vi "外控留样模式参数.vi"() -> ()   [LabVIEW 2016, in "超标留样集成.lvlib" / "德润DR803M超标留样.lvlib"]
uses:
  <vilib>/Utility/miscctls.llb/LVPointTypeDef.ctl
panel:
  out "读取更新":bool
  in  "返回":bool
  in  "模拟设置":bool
  in  "每瓶次数：":dbl
  in  "平行样：":dbl
  in  "每次留样：":dbl
  in  "留样瓶数：":dbl
  in  "当前瓶号：":dbl
  # "在该画面下，可设置该模式下的采样参数，包括当前瓶号、平行样、留样瓶数、每瓶次数和每次留样量。"
  # "mL"
  # "mg/L"
  # "COD\n模拟\n设置"
  # "mg/L"
  # "mg/L"
  # "mg/L"
  # "mg/L"
  # "氨氮\n模拟\n设置"
  # "mg/L"
  # "mg/L"
  # "mg/L"
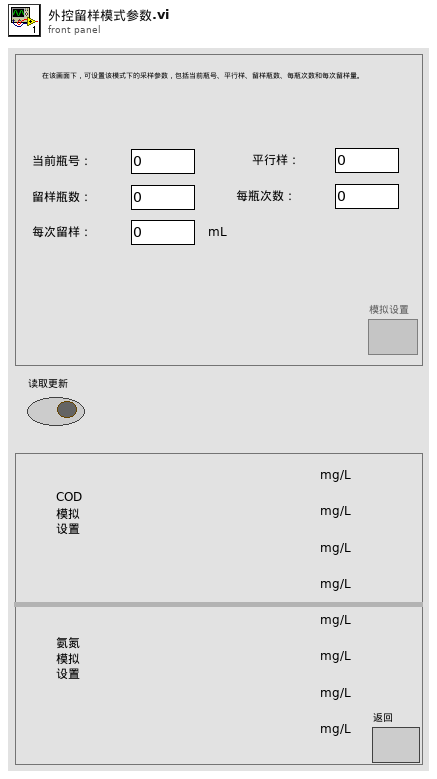
[diagram p1: front panel]
types:
  T1 = typedef "LVPointTypeDef.ctl" = cluster{"Horizontal":i16, "Vertical":i16}
  T2 = cluster{"当前瓶号：":dbl, "平行样：":dbl, "留样瓶数：":dbl, "每瓶次数：":dbl, "每次留样：":dbl}
  T3 = cluster{"采样器状态":enum16{"停止", "运行", "系统初始化-2", "系统初始化-3", "初始化失败"}, "仪器时间":timestamp, "留样结果":bool, "工作模式":u16, "当前瓶号":u16, "平行样数":u16, "采样瓶数":u16, "设定每瓶采样次数":u16, "每瓶采样量":u16, "当前进程":u16, "当前瓶已采次数":u16, "留样中":bool}
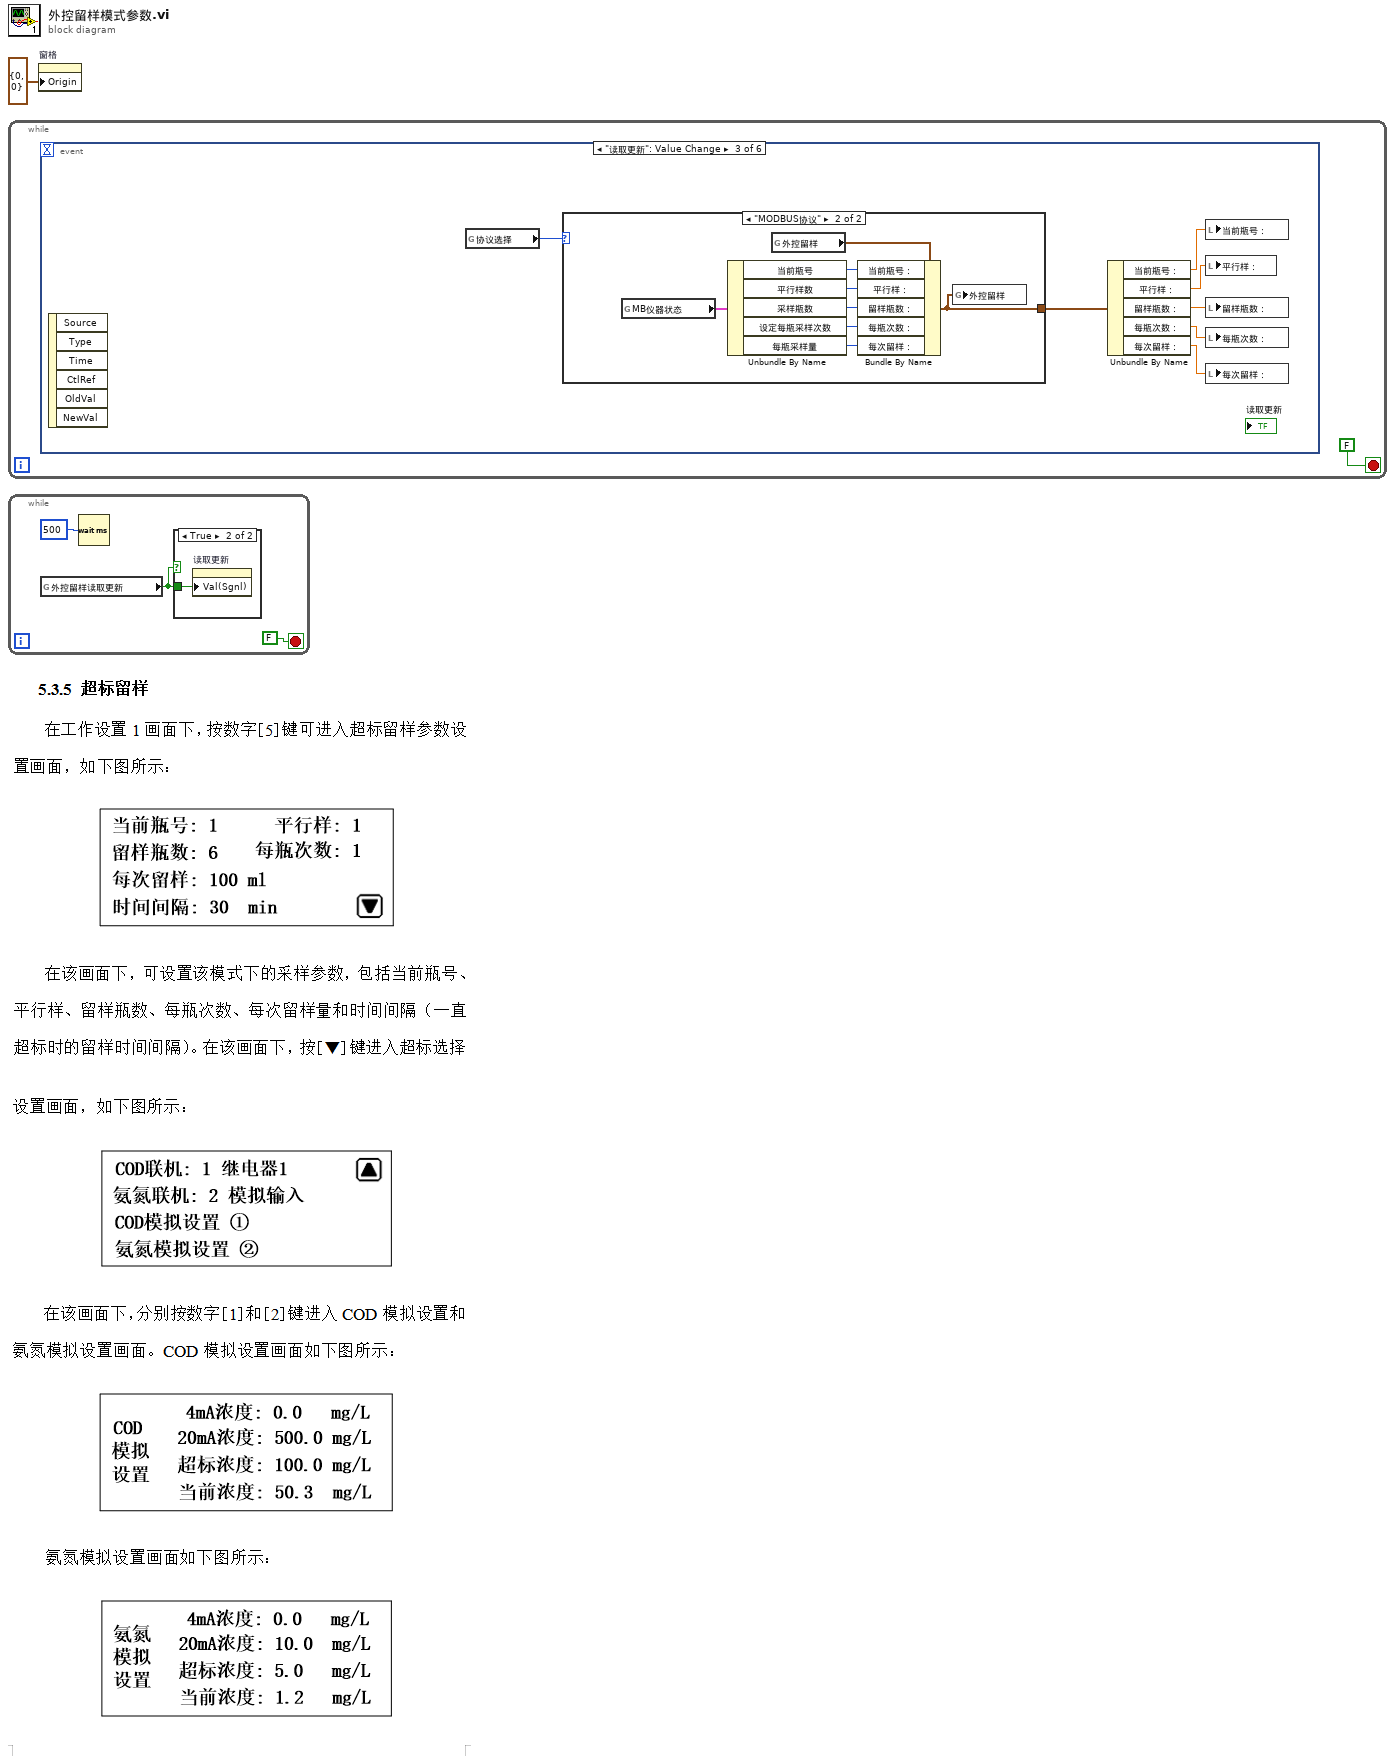
[diagram p0: block diagram]
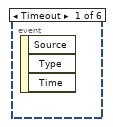
[diagram p2: hidden frame]
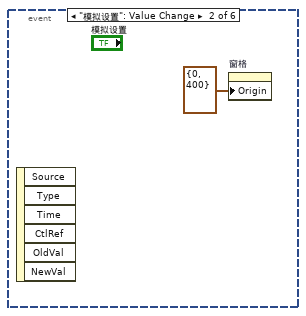
[diagram p3: hidden frame]
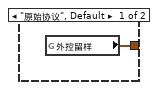
[diagram p4: hidden frame]
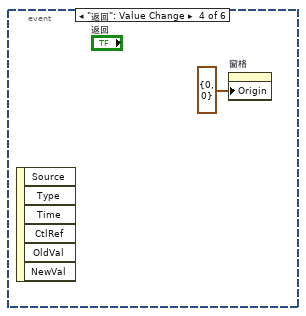
[diagram p5: hidden frame]
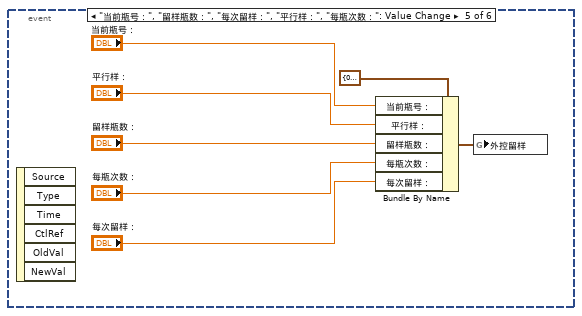
[diagram p6: hidden frame]
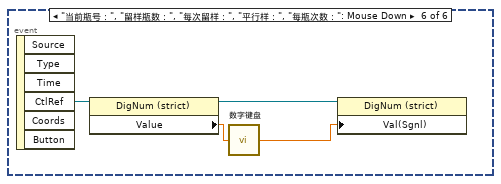
[diagram p7: hidden frame]
diagram:
  n1 = while {
    stop <- FALSE stop-if-true
    n2 = event shown="[2] \"读取更新\": Value Change" {
      selector: _ -> [_ _ _ _ _ _]
      dyn-events: _ -> [_ _ _ _ _ _]
      timeout: _ -> [_ _ _ _ _ _]
      event Timeout {
        n3 = event-data() -> ()  [unwired: 1 in, 3 out]
      }
      event "模拟设置": Value Change {
        n4 = event-data() -> ()  [unwired: 1 in, 6 out]
        n5 = property on="窗格" class="Pane"("Origin"=T1 {"Horizontal"=0, "Vertical"=400} ("原点")) -> ()  [unwired: 2 in, 2 out]
      }
      event "读取更新": Value Change {
        n6 = event-data() -> ()  [unwired: 1 in, 6 out]
        n7 = global read "超标留样全局.vi" "协议选择"() -> (w4:enum16{"原始协议", "MODBUS协议"})
        n8 = case shown="\"MODBUS协议\"" w4 {
          tunnel: [w11 w12] -> w5
          frame "原始协议", Default {
            n9 = global read "超标留样全局.vi" "外控留样"() -> (w11:T2)
          }
          frame "MODBUS协议" {
            n10 = global read "超标留样全局.vi" "MB仪器状态"() -> (w19:T3)
            n11 = Unbundle By Name(w19) -> ("当前瓶号"=w17:u16, "平行样数"=w16:u16, "采样瓶数"=w15:u16, "设定每瓶采样次数"=w14:u16, "每瓶采样量"=w13:u16)
            n12 = global read "超标留样全局.vi" "外控留样"() -> (w18:T2)
            n13 = Bundle By Name(cluster=w18, "当前瓶号："=w17, "平行样："=w16, "留样瓶数："=w15, "每瓶次数："=w14, "每次留样："=w13) -> (w12:T2)
            n14 = global write "超标留样全局.vi" "外控留样"(w12) -> ()
          }
        }
        n15 = Unbundle By Name(w5) -> ("当前瓶号："=w10:dbl, "平行样："=w9:dbl, "留样瓶数："=w8:dbl, "每瓶次数："=w7:dbl, "每次留样："=w6:dbl)
        n16 = local write "当前瓶号："(w10) -> ()
        n17 = local write "平行样："(w9) -> ()
        n18 = local write "留样瓶数："(w8) -> ()
        n19 = local write "每瓶次数："(w7) -> ()
        n20 = local write "每次留样："(w6) -> ()
      }
      event "返回": Value Change {
        n21 = event-data() -> ()  [unwired: 1 in, 6 out]
        n22 = property on="窗格" class="Pane"("Origin"=T1 {"Horizontal"=0, "Vertical"=0} ("原点")) -> ()  [unwired: 2 in, 2 out]
      }
      event "当前瓶号：", "留样瓶数：", "每次留样：", "平行样：", "每瓶次数：": Value Change {
        n23 = event-data() -> ()  [unwired: 1 in, 6 out]
        n24 = Bundle By Name(cluster=T2 {"当前瓶号："=0.0, "平行样："=0.0, "留样瓶数："=0.0, "每瓶次数："=0.0, "每次留样："=0.0} ("外控留样"), "当前瓶号："="当前瓶号：", "平行样："="平行样：", "留样瓶数："="留样瓶数：", "每瓶次数："="每瓶次数：", "每次留样："="每次留样：") -> (w21:T2)
        n25 = global write "超标留样全局.vi" "外控留样"(w21) -> ()
      }
      event "当前瓶号：", "留样瓶数：", "每次留样：", "平行样：", "每瓶次数：": Mouse Down {
        n26 = event-data() -> ("CtlRef"=w31:refnum<vi>)  [unwired: 1 in, 5 out]
        n27 = property class="DigNum (strict)"(reference=w31) -> (reference out=w29:refnum<vi>, "Value"=w30:dbl)  [unwired: 1 in, 1 out]
        n28 = call "数字键盘.vi"("OldNumber"=w30) -> ("NewNumber"=w28:sgl)
        n29 = property class="DigNum (strict)"(reference=w29, "Val(Sgnl)"=w28) -> ()  [unwired: 1 in, 2 out]
      }
    }
  }
  n30 = while {
    stop <- FALSE stop-if-true
    n31 = global read "超标留样全局.vi" "外控留样读取更新"() -> (w32:bool)
    n32 = Wait (ms)(milliseconds to wait=u32 500 ("等待时间（毫秒）")) -> ()  [unwired: 1 out]
    n33 = case shown="True" w32 {
      tunnel: w32 -> [_ w35]
      frame False {
      }
      frame True {
        n34 = property on="读取更新" class="Bool (strict)"("Val(Sgnl)"=w35) -> ()  [unwired: 2 in, 2 out]
      }
    }
  }
  n35 = property on="窗格" class="Pane"("Origin"=T1 {"Horizontal"=0, "Vertical"=0} ("原点")) -> ()  [unwired: 2 in, 2 out]
